vi "String to boolean.vi"(11 "String":string) -> (3 "Boolean":bool)   [LabVIEW 2013]
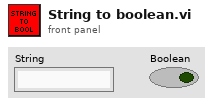
[diagram p1: front panel]
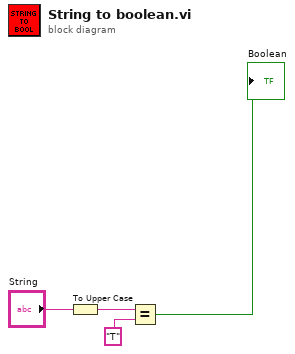
[diagram p0: block diagram]
diagram:
  n1 = To Upper Case(1:"String") -> (0:w2:string)
  n2 = Equal?(x=w2, y="T") -> (x = y?=→"Boolean":bool)
